vi "Search.vi"(8 "error in (no error)":errorcluster, 10 "GraphNode in":refnum<data-value>, 11 "GraphSearch in":refnum<class "GraphSearch.lvclass">) -> (0 "error out":errorcluster, 1 "found":bool, 2 "GraphNode out":refnum<data-value>, 3 "GraphSearch out":refnum<class "GraphSearch.lvclass">, 4 "Path":refnum<data-value>[](array[refnum]))   [LabVIEW 2009, in "GraphSearch.lvclass"]
uses:
  GraphSearch.lvclass
  GraphNode/GraphNode.lvclass
  GraphSearch.lvclass/GraphSearch.ctl
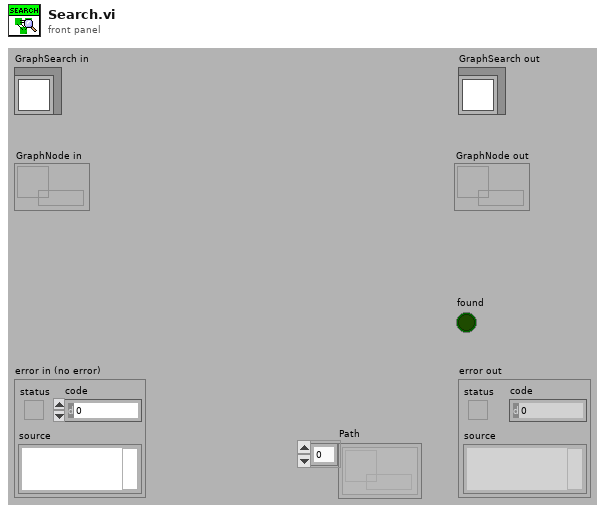
[diagram p1: front panel]
types:
  T1 = typedef "GraphSearch.lvclass/method.ctl" = enum16{"Breadth", "Heuristic", "Depth"}
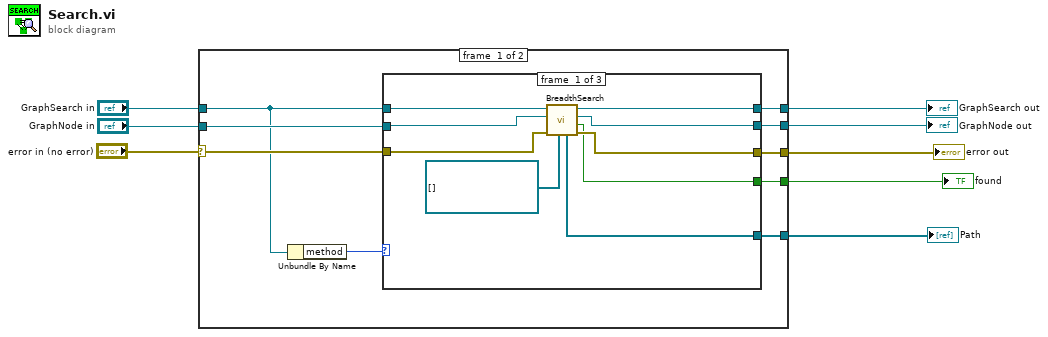
[diagram p0: block diagram]
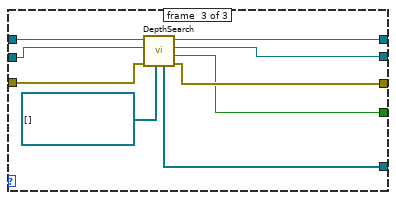
[diagram p3: hidden frame]
diagram:
  n1 = case shown="No Error" "error in (no error)" {
    selector: "error in (no error)" -> [w14 w41]
    tunnel: [w13 w41] -> w7
    tunnel: [w15 w40] -> w5
    tunnel: "GraphSearch in" -> [w10 w40]
    tunnel: "GraphNode in" -> [w17 w39]
    tunnel: [w16 w39] -> w3
    tunnel: [w12 _] -> w2
    tunnel: [w11 _] -> w1
    frame #0 {
      n2 = Unbundle By Name(w10) -> ("method"=w9:T1)
      n3 = case shown="\"Breadth\", Default" w9 {
        tunnel: w10 -> [w26 w29 w38]
        tunnel: w17 -> [w24 w28 w37]
        tunnel: [w23 w28 w36] -> w16
        tunnel: [w25 w29 w35] -> w15
        tunnel: w14 -> [w22 w27 w34]
        tunnel: [w21 w27 w33] -> w13
        tunnel: [w20 _ w32] -> w12
        tunnel: [w19 _ w31] -> w11
        frame #0 {
          n4 = call "BreadthSearch.vi"("Path in"=refnum<data-value>[] [], "error in (no error)"=w22, "GraphNode in"=w24, "GraphSearch in"=w26) -> ("error out"=w21:errorcluster, "found"=w19:bool, "GraphNode out"=w23:refnum<data-value>, "GraphSearch out"=w25:refnum<class "GraphSearch.lvclass">, "Path out"=w20:refnum<data-value>[])  [unwired: 3 in]
        }
        frame #1 {
        }
        frame #2 {
          n5 = call "DepthSearch.vi"("Path in"=refnum<data-value>[] [], "error in (no error)"=w34, "GraphNode in"=w37, "GraphSearch in"=w38) -> ("error out"=w33:errorcluster, "found"=w31:bool, "GraphNode out"=w36:refnum<data-value>, "GraphSearch out"=w35:refnum<class "GraphSearch.lvclass">, "Path out"=w32:refnum<data-value>[])  [unwired: 3 in]
        }
      }
    }
    frame #1 {
    }
  }
  "error out" <- w7
  "GraphSearch out" <- w5
  "GraphNode out" <- w3
  "found" <- w1
  "Path" <- w2
